vi "UTILITY Debug Search Parameters.vi"(6 "File Locations In":T1, 8 "Error In":errorcluster, 10 "all rows":string[][](array[string])) -> (0 "Error Out":errorcluster)   [LabVIEW 2016]
uses:
  Save File/File Setup (Public)/Type Definition/Save File DOE File Path Control.ctl
  Save File/File Setup (Public)/Type Definition/Save File DOE Data Save Filepaths.ctl
  Type Definitions/UTILITY Default File Create.ctl
  Save File/Save File.lvlib
  Save File/File Setup.lvlib
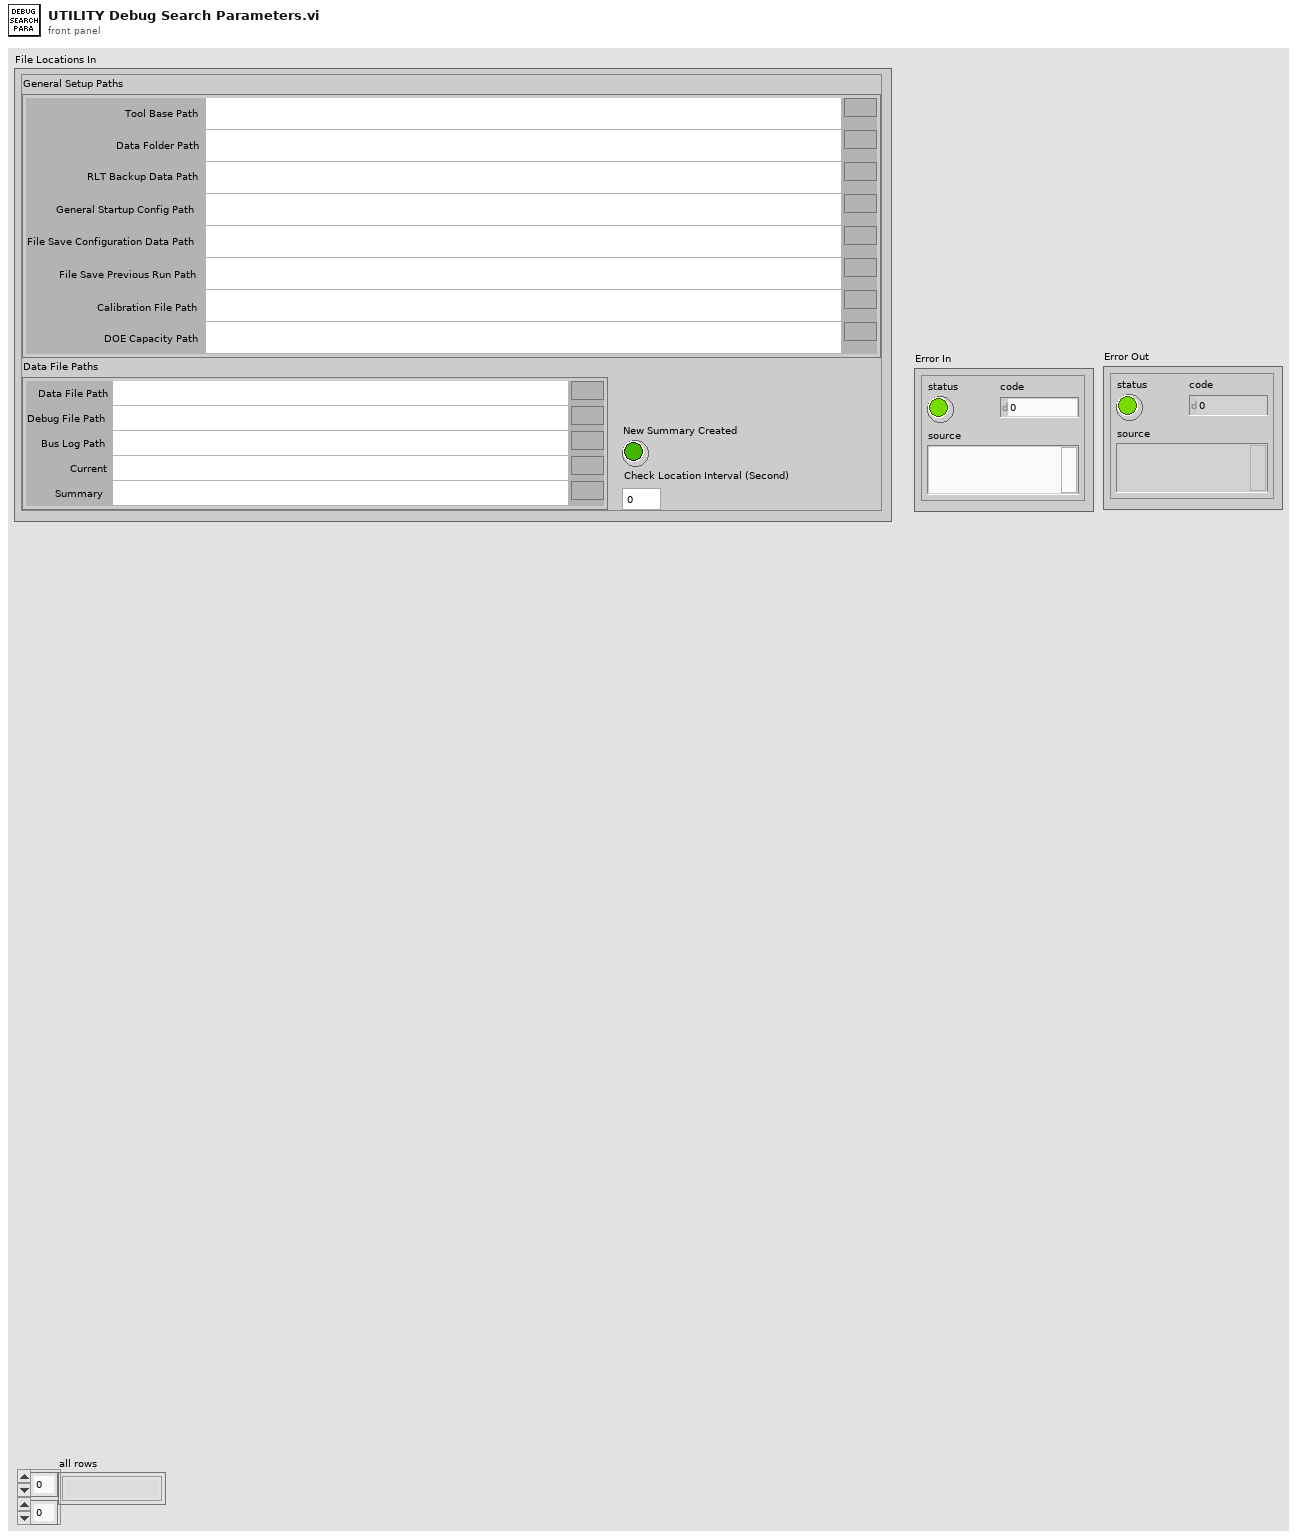
[diagram p1: front panel]
types:
  T1 = typedef "File Setup.lvlib/Save File DOE File Path Control.ctl" = cluster{"General Setup Paths":cluster{"Calibration File Path":path, "DOE Capacity Path":path, "Data Folder Path":path, "RLT Backup Data Path":path, "Tool Base Path":path, "General Startup Config Path":path, "File Save Previous Run Path":path, "File Save Configuration Data Path":path}, "Data File Paths":T2, "New Summary Created":bool, "Check Location Interval (Second)":i32}
  T2 = typedef "File Setup.lvlib/Save File DOE Data Save Filepaths.ctl" = cluster{"Data File Path":path, "Debug File Path":path, "Bus Log Path":path, "Current":path, "Summary":path}
  T3 = typedef "UTILITY Default File Create.ctl" = enum16{"Configuration File", "Debug Search File", "WILT Water Injection Times", "WILT Agilent Assignment", "WILT Save Status Path", "WILT General Config"}
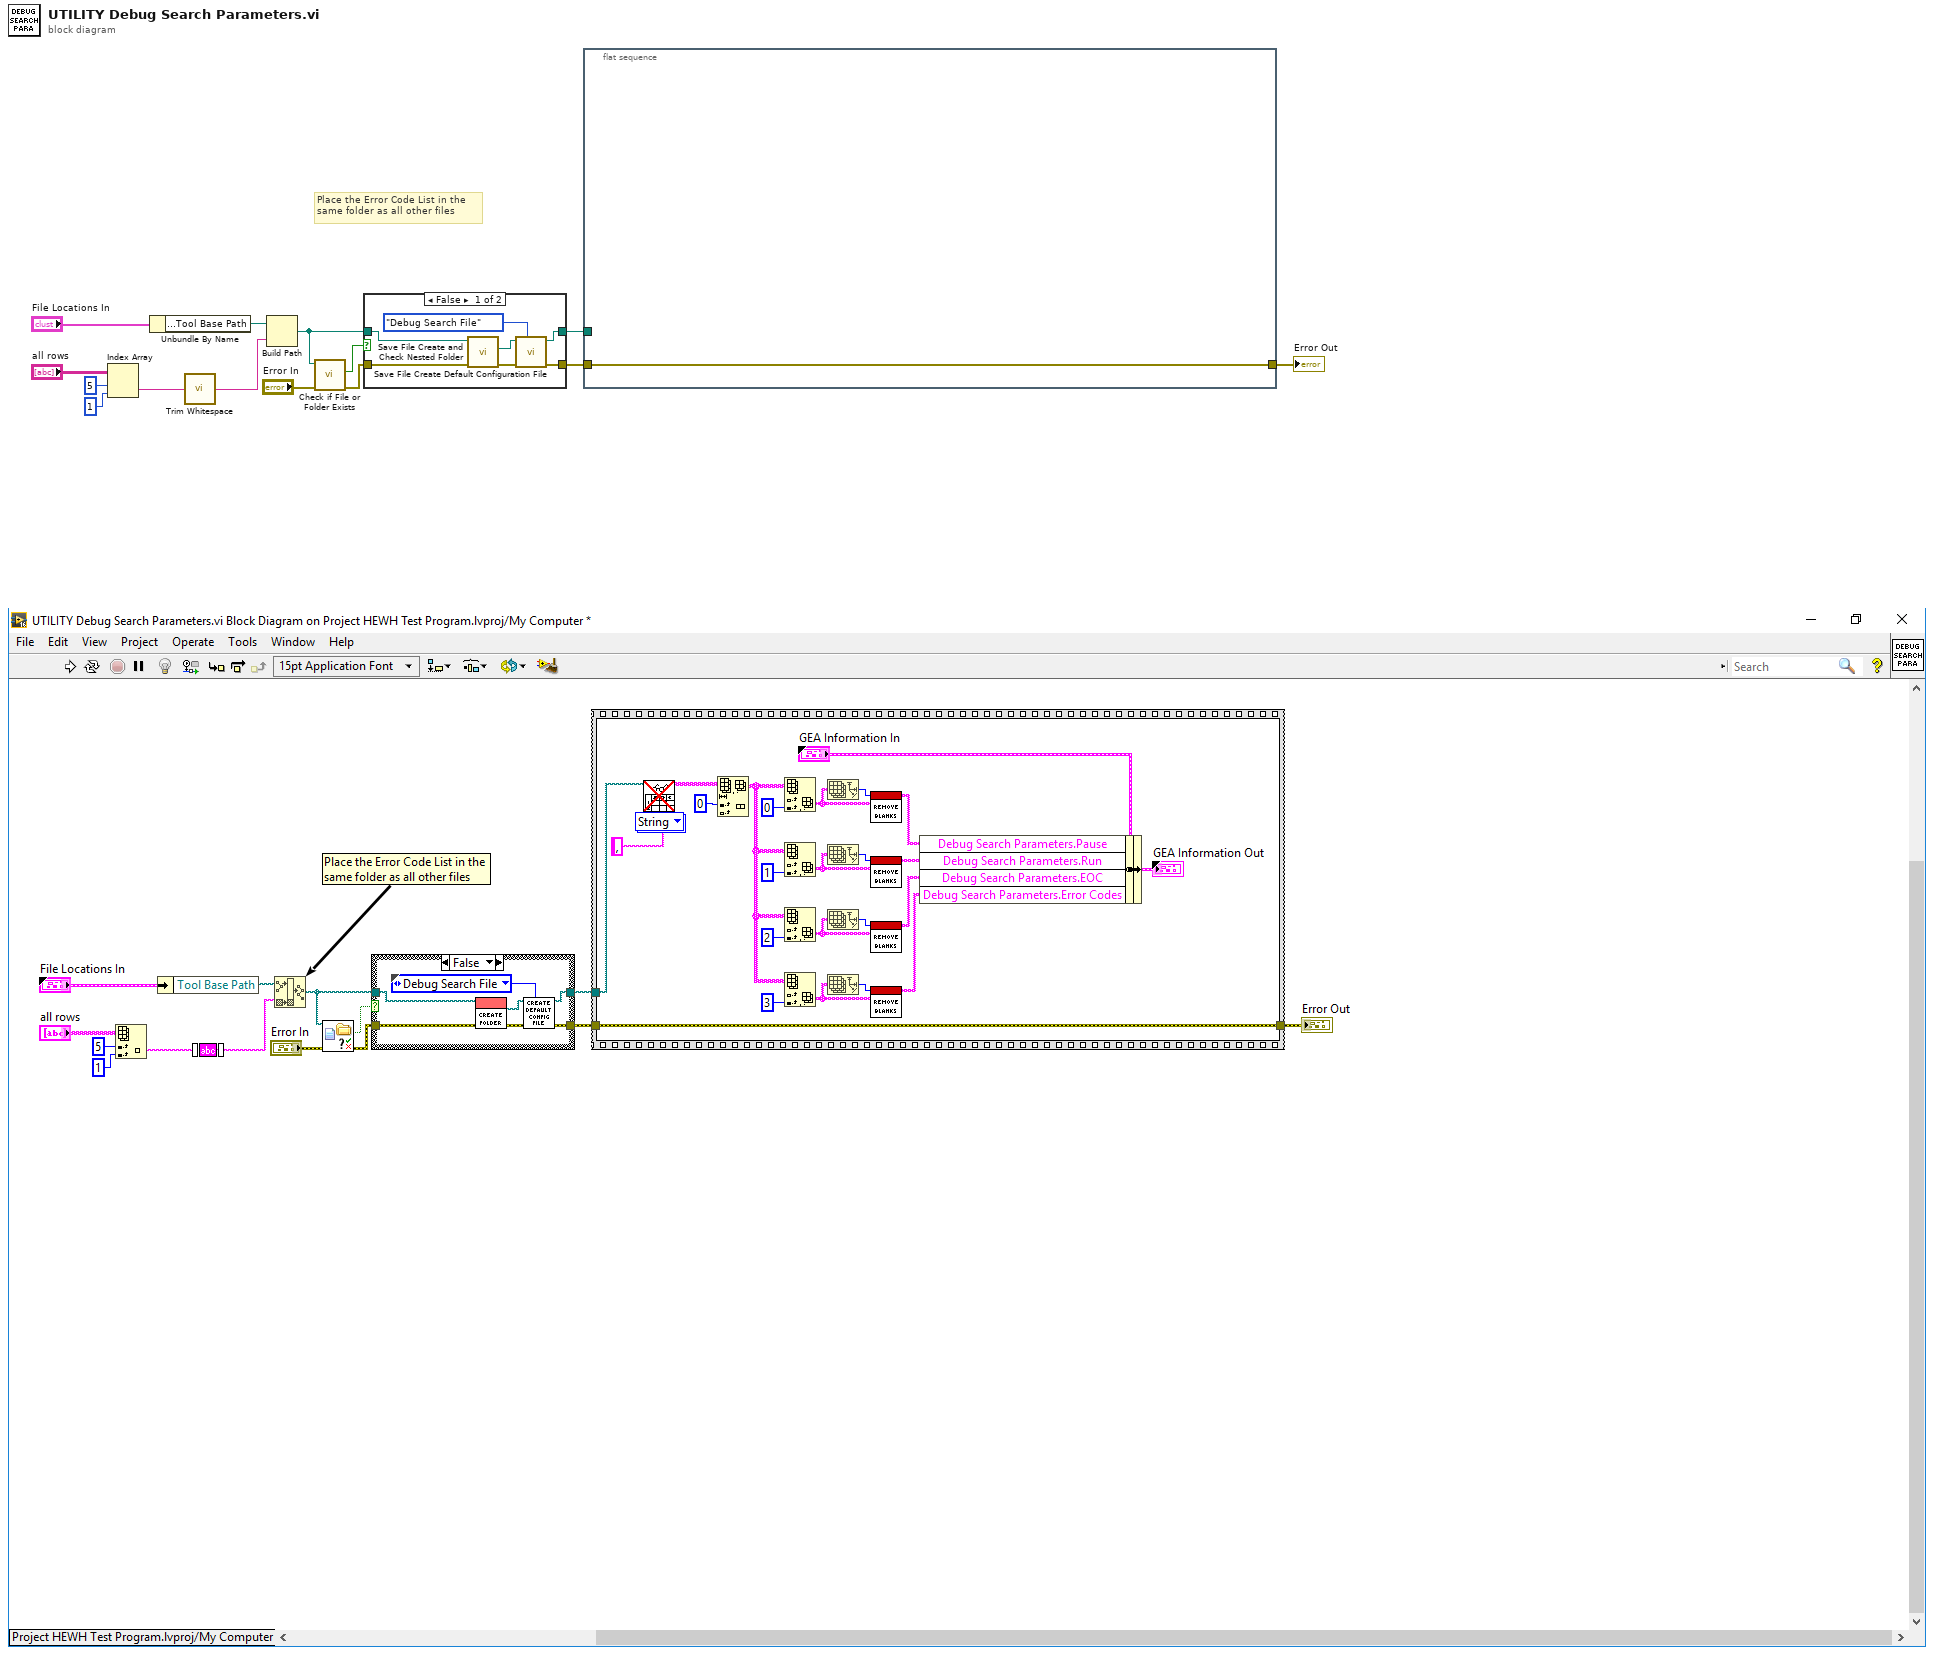
[diagram p0: block diagram]
diagram:
  # "Place the Error Code List in the \nsame folder as all other files"
  n1 = Index Array(array="all rows", index (row)=5, index (col)=1) -> (element=w13:string)
  n2 = Unbundle By Name("File Locations In") -> ("General Setup Paths.Tool Base Path"=w3:path)
  n3 = call <vilib>:"Trim Whitespace.vi"("string"=w13) -> ("trimmed string"=w2:string)  [unwired: 1 in]
  n4 = Build Path(base path=w3, name or relative path=w2) -> (appended path=w1:path)
  n5 = call <vilib>:"Check if File or Folder Exists.vi"("error in (no error)"="Error In", "path"=w1) -> ("error out"=w8:errorcluster, "file or folder exists?"=w10:bool)  [unwired: 7 in, 1 out]
  n6 = case shown="False" w10 {
    tunnel: w1 -> [w21 w23]
    tunnel: [w17 w23] -> w5
    tunnel: w8 -> [w20 w22]
    tunnel: [w18 w22] -> w7
    frame False {
      n7 = call "Save File Create and Check Nested Folder.vi"("error in (no error)"=w20, "Extracted File Name"=w21) -> ("error out"=w19:errorcluster, "File Path"=w16:path)  [unwired: 7 in, 1 out]
      n8 = call "Save File Create Default Configuration File.vi"("Default File Create"=UTILITY_Default_File_Create."Debug Search File", "Error In"=w19, "File Path In"=w16) -> ("Error Out"=w18:errorcluster, "File Path Out"=w17:path)  [unwired: 7 in]
    }
    frame True {
    }
  }
  n9 = flat-sequence {
    tunnel: w5 -> [_]
    tunnel: w7 -> [w24]
    tunnel: [w24] -> w6
    frame #0 {
    }
  }
  "Error Out" <- w6
